vi "xiC - IMAQ - RebuildTree.vi"(6 "TreeItems[]":T1(array[cluster]), 8 "error in (no error)":errorcluster, 11 "Attributes":T2) -> (0 "error out":errorcluster, 3 "Attributes":T2)   [LabVIEW 2013]
uses:
  xiC - IMAQ - Attributes.ctl
  C:/Projects/Cameras3.x/xiLib/xiLIB_64bit/xiLIB/xiCamLib/API/x64/xiApi.NETX64.dll
  xiLIB_64bit/xiLIB/xiCamLib/API/x64/xiApi.NETX64.dll
  xiC - IMAQ - TreeDisplayType.ctl
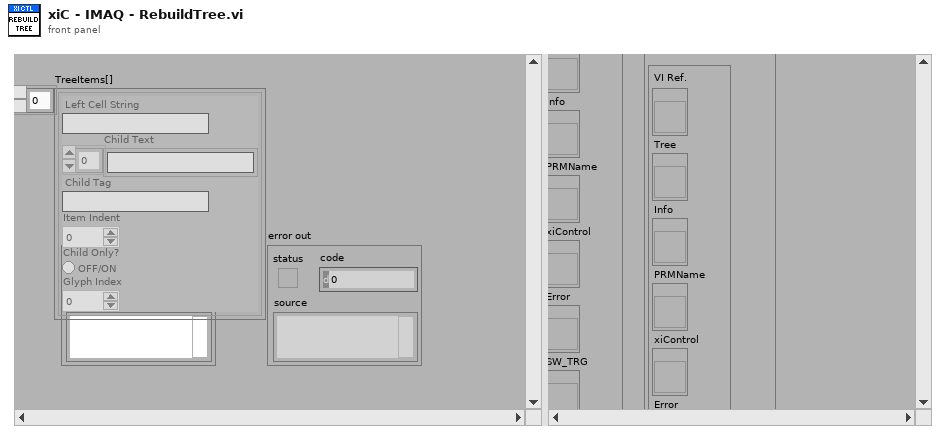
[diagram p1: front panel]
types:
  T1 = cluster{"Left Cell String":string, "Child Text":string[], "Child Tag":string, "Item Indent":i32, "Child Only?":bool, "Glyph Index":i32}[]
  T2 = typedef "xiC - IMAQ - Attributes.ctl" = cluster{"Controls":cluster{"VI Ref.":refnum<vi>, "Tree":refnum<vi>, "Info":refnum<vi>, "PRMName":refnum<vi>, "xiControl":refnum<vi>, "Error":refnum<vi>, "SW_TRG":refnum<vi>, "ImageDisplay":refnum<vi>}, "Variables":cluster{"ProcessQ.":refnum<queue>, "Data":bool, "xiCam":refnum<k24>, "Tree_Display_Type":T3}}
  T3 = typedef "xiC - IMAQ - TreeDisplayType.ctl" = enum16{"DEFAULT", "HIDE_MAX_MIN"}
  T4 = typedef "LVNodeAndColumnTypeDef.ctl" = cluster{"Node":string, "Column":i32}
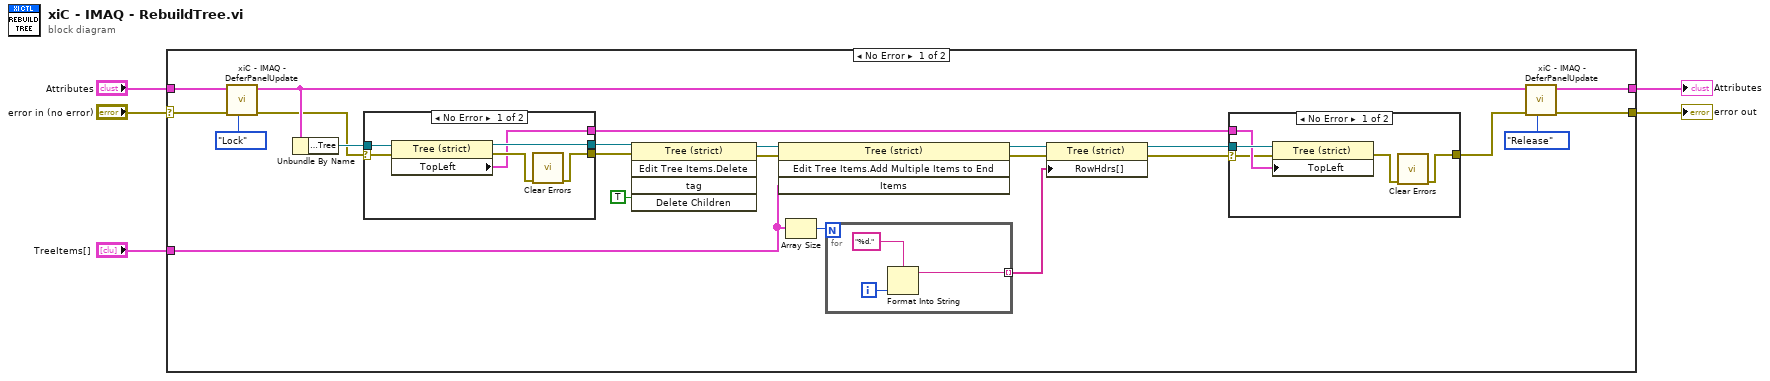
[diagram p0: block diagram]
diagram:
  n1 = case shown="No Error" "error in (no error)" {
    selector: "error in (no error)" -> [w22 w47]
    tunnel: [w23 w47] -> w4
    tunnel: "Attributes" -> [w21 w46]
    tunnel: [w20 w46] -> w2
    tunnel: "TreeItems[]" -> [w7 _]
    frame No Error {
      n2 = call "xiC - IMAQ - DeferPanelUpdate.vi"("Operand"=enum16{"Lock", "Release"}."Lock", "error in (no error)"=w22, "Attributes"=w21) -> ("error out"=w15:errorcluster, "Attributes"=w19:T2)  [unwired: 7 in]
      n3 = Unbundle By Name(w19) -> ("Controls.Tree"=w16:refnum<vi>)
      n4 = case shown="No Error" w15 {
        selector: w15 -> [w36 w39]
        tunnel: w16 -> [w37 w38]
        tunnel: [w34 w39] -> w14
        tunnel: [w33 w38] -> w13
        tunnel: [w32 _] -> w12
        frame No Error {
          n5 = property class="Tree (strict)"(reference=w37, error in=w36) -> (reference out=w33:refnum<vi>, error out=w35:errorcluster, "TopLeft"=w32:T4)
          n6 = call <vilib>:"Clear Errors.vi"("error in (no error)"=w35) -> ("error out"=w34:errorcluster)  [unwired: 6 in]
        }
        frame Error {
        }
      }
      n7 = invoke class="Tree (strict)" method="Edit Tree Items.Delete"(reference=w13, error in=w14, "Delete Children"=TRUE ("Delete Children?")) -> (reference out=w26:refnum<vi>, error out=w25:errorcluster)  [unwired: 2 in, 3 out]
      n8 = invoke class="Tree (strict)" method="Edit Tree Items.Add Multiple Items to End"(reference=w26, error in=w25, "Items"=w7) -> (reference out=w18:refnum<vi>, error out=w10:errorcluster)  [unwired: 1 in, 2 out]
      n9 = Array Size(array=w7) -> (size(s)=w8:i32)
      n10 = for {
        N: w8 -> [_]
        tunnel: [w29] -> w6 mode=indexing
        i -> [w31]
        n11 = Format Into String(format string="%d.", w31) -> (resulting string=w29:string)  [unwired: 2 in, 1 out]
      }
      n12 = property class="Tree (strict)"(reference=w18, error in=w10, "RowHdrs[]"=w6) -> (reference out=w11:refnum<vi>, error out=w9:errorcluster)
      n13 = case shown="No Error" w9 {
        selector: w9 -> [w42 w45]
        tunnel: w11 -> [w44 _]
        tunnel: w12 -> [w43 _]
        tunnel: [w40 w45] -> w17
        frame No Error {
          n14 = property class="Tree (strict)"(reference=w44, error in=w42, "TopLeft"=w43) -> (error out=w41:errorcluster)  [unwired: 1 out]
          n15 = call <vilib>:"Clear Errors.vi"("error in (no error)"=w41) -> ("error out"=w40:errorcluster)  [unwired: 6 in]
        }
        frame Error {
        }
      }
      n16 = call "xiC - IMAQ - DeferPanelUpdate.vi"("Operand"=enum16{"Lock", "Release"}."Release", "error in (no error)"=w17, "Attributes"=w19) -> ("error out"=w23:errorcluster, "Attributes"=w20:T2)  [unwired: 7 in]
    }
    frame Error {
    }
  }
  "error out" <- w4
  "Attributes" <- w2
